vi "Add Multiple Headers.vi"(8 "error in":errorcluster, 10 "Headers":refnum<class "httpHeaders.lvclass">, 11 "http-client in":refnum<class "httpClient.lvclass">) -> (0 "error out":errorcluster, 3 "http-client out":refnum<class "httpClient.lvclass">)   [LabVIEW 2020, in "httpClient.lvlib" / "httpClient.lvclass"]
uses:
  httpClient.lvclass
  httpHeaders/httpHeaders.lvclass
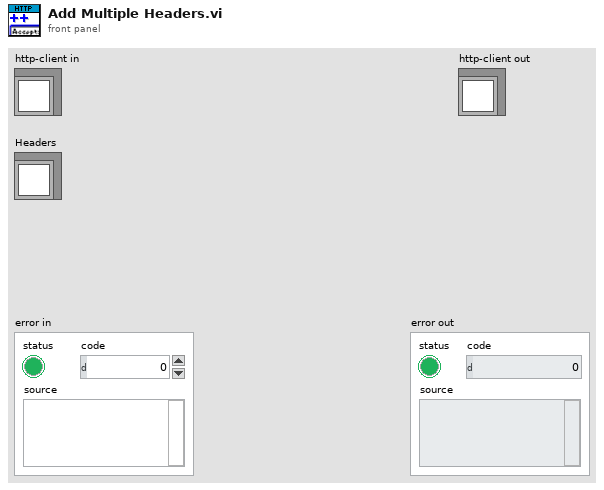
[diagram p1: front panel]
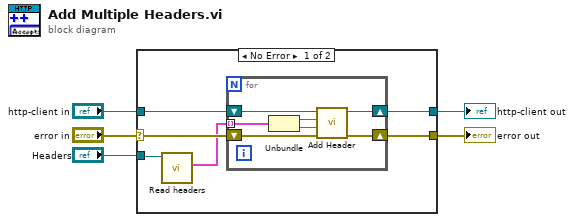
[diagram p0: block diagram]
diagram:
  n1 = case shown="No Error" "error in" {
    selector: "error in" -> [w10 w20]
    tunnel: [w9 w20] -> w4
    tunnel: [w8 w19] -> w2
    tunnel: "http-client in" -> [w11 w19]
    tunnel: "Headers" -> [w6 _]
    frame No Error {
      n2 = call "Read headers.vi"("httpHeaders in"=w6) -> ("headers"=w7:cluster{"header":string, "value":string}[])  [unwired: 8 in, 2 out]
      n3 = for {
        shift-right: [w12] -> w9
        shift-left: w10 -> [w13]
        shift-right: [w16] -> w8
        shift-left: w11 -> [w17]
        tunnel: w7 -> [w18] mode=indexing
        n4 = Unbundle(w18) -> ("header"=w15:string, "value"=w14:string)
        n5 = call "Add Header.vi"("error in"=w13, "value"=w14, "header"=w15, "http-client in"=w17) -> ("error out"=w12:errorcluster, "http-client out"=w16:refnum<class "httpClient.lvclass">)  [unwired: 6 in]
      }
    }
    frame Error {
    }
  }
  "error out" <- w4
  "http-client out" <- w2
